vi "Check-Out.vi"(8 "error in (no error)":errorcluster, 9 "Timeout (-1)":dbl[unit], 11 "Object Reference":refnum<class "CS++Reference.lvclass">) -> (0 "error out":errorcluster, 1 "Object valid??":bool, 2 "Object":refnum<class "CS++Base.lvclass">, 3 "Object Reference out":refnum<class "CS++Reference.lvclass">)   [LabVIEW 2016, in "CS++BaseClasses.lvlib" / "CS++Reference.lvclass"]
doc: "Checkout object from Reference."
uses:
  CS++Reference.lvclass
  Base/CS++Base.lvclass
  CS++Reference.lvclass/CS++Reference.ctl
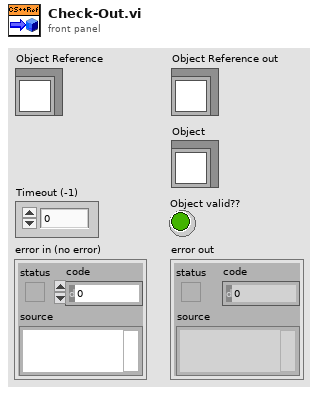
[diagram p1: front panel]
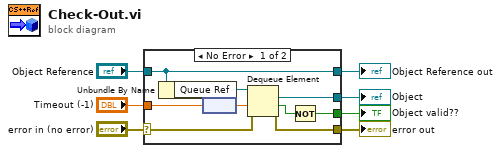
[diagram p0: block diagram]
diagram:
  n1 = case shown="No Error" "error in (no error)" {
    selector: "error in (no error)" -> [w14 w18]
    tunnel: [w11 w18] -> w6
    tunnel: [w16 w17] -> w4
    tunnel: "Object Reference" -> [w16 w17]
    tunnel: "Timeout (-1)" -> [w12 _]
    tunnel: [w10 _] -> w2
    tunnel: [w8 _] -> w1
    frame No Error {
      n2 = Unbundle By Name(w16) -> ("Queue Ref"=w15:refnum<queue>)
      n3 = node(w12) -> (w13:dbl)
      n4 = Dequeue Element(queue=w15, timeout in ms (-1)=w13, error in (no error)=w14) -> (element=w10:refnum<class "CS++Base.lvclass">, timed out?=w9:bool, error out=w11:errorcluster)  [unwired: 1 out]
      n5 = Not(x=w9) -> (.not. x?=w8:bool)
    }
    frame Error {
    }
  }
  "error out" <- w6
  "Object Reference out" <- w4
  "Object" <- w2
  "Object valid??" <- w1
